vi "Is Valid.vi"(8 "error in (no error)":errorcluster, 11 "Transfer Configuration in":refnum<class "Configuration.Transfer.lvclass">) -> (0 "error out":errorcluster, 1 "invalid channel indicies":i32[](array[numeric]), 2 "valid?":bool, 3 "Transfer Configuration out":refnum<class "Configuration.Transfer.lvclass">)   [LabVIEW 2016, in "Data Sharing Framework.Configuration.lvlib" / "Configuration.Transfer.lvclass"]
uses:
  Configuration.Transfer.lvclass
  Configuration.Transfer.lvclass/Configuration.Transfer.ctl
  Configuration.Channel/Configuration.Channel.lvclass/Configuration.Channel.ctl
  Configuration.Channel/Configuration.Channel.lvclass
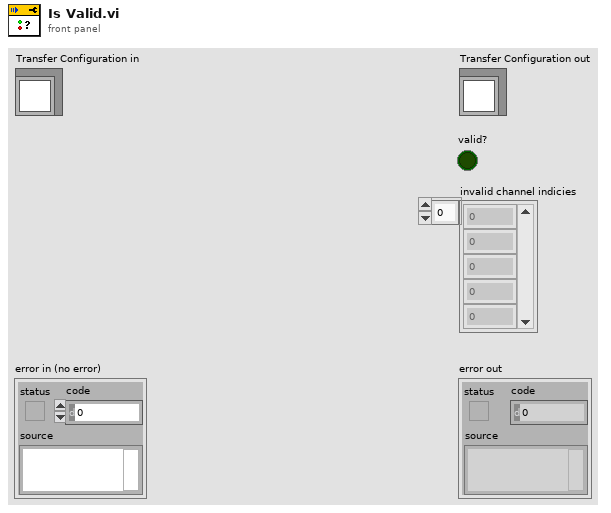
[diagram p1: front panel]
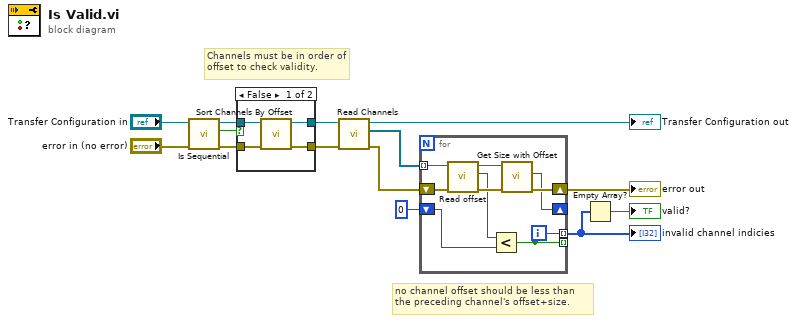
[diagram p0: block diagram]
diagram:
  # "no channel offset should be less than the preceding channel's offset+size."
  # "Channels must be in order of offset to check validity."
  n1 = call "Is Sequential.vi"("error in (no error)"="error in (no error)", "Transfer Configuration in"="Transfer Configuration in") -> ("error out"=w7:errorcluster, "sequential offsets?"=w8:bool, "Transfer Configuration out"=w9:refnum<class "Configuration.Transfer.lvclass">)  [unwired: 7 in]
  n2 = case shown="False" w8 {
    tunnel: [w18 w20] -> w14
    tunnel: [w17 w19] -> w13
    tunnel: w9 -> [w16 w20]
    tunnel: w7 -> [w15 w19]
    frame False {
      n3 = call "Sort Channels By Offset.vi"("error in (no error)"=w15, "Transfer Configuration in"=w16) -> ("error out"=w17:errorcluster, "Transfer Configuration out"=w18:refnum<class "Configuration.Transfer.lvclass">)  [unwired: 8 in]
    }
    frame True {
    }
  }
  n4 = call "Read Channels.vi"("error in (no error)"=w13, "Configuration.Transfer in"=w14) -> ("error out"=w5:errorcluster, "Channels"=w12:refnum<class "Configuration.Channel.lvclass">[], "Configuration.Transfer out"=→"Transfer Configuration out":refnum<class "Configuration.Transfer.lvclass">)  [unwired: 7 in]
  n5 = for {
    tunnel: w12 -> [w30] mode=indexing
    shift-right: [w28] -> w4
    shift-left: w5 -> [w27]
    tunnel: [w24] -> w3 mode=indexing if=w23
    tunnel: [w23] -> _ mode=indexing
    shift-right: [w21] -> _
    shift-left: u64 0 ("size+offset in bytes") -> [w22]
    i -> [w24]
    n6 = call "Read offset.vi"("error in (no error)"=w27, "Configuration.Channel in"=w30) -> ("error out"=w26:errorcluster, "offset"=w25:u64, "Configuration.Channel out"=w29:refnum<class "Configuration.Channel.lvclass">)  [unwired: 7 in]
    n7 = Less?(x=w25, y=w22) -> (x < y?=w23:bool)
    n8 = call "Get Size with Offset.vi"("error in (no error)"=w26, "Channel Configuration in"=w29) -> ("error out"=w28:errorcluster, "size+offset in bytes"=w21:u64)  [unwired: 7 in, 1 out]
  }
  "error out" <- w4
  "invalid channel indicies" <- w3
  n9 = Empty Array?(array=w3) -> (empty?=→"valid?":bool)
